vi "Dataset_Reader(Classification).vi"(3 "Train dataset path":path=path "D:/working/Anomaly Detection/Train") -> (0 "error out":errorcluster, 1 "Dataset":T1)   [LabVIEW 2020]
uses:
  <vilib>/Ngene/DeepLTK/Toolkit/NN_Data/API/DataSet_Types/NN_DataSet(In1D_Out1D).ctl
  <vilib>/Ngene/DeepLTK/Toolkit/NN_Data/API/DataRef_Types/NN_Data_ref(2D_SGL).ctl
  <vilib>/Ngene/DeepLTK/Toolkit/NN_Data/API/DataRef_Types/NN_Data_ref(1D_I32).ctl
  8703a7eb-7e7a-4f89-999d-626aab8b5f58.vi
  <vilib>/Utility/file.llb/Read Delimited Spreadsheet (DBL).vi
  <vilib>/Comparison/Less/Less Functor/Less Functor.lvclass
  <vilib>/Ngene/DeepLTK/Toolkit/Deep_Learning_Toolkit_by_Ngene.lvlib
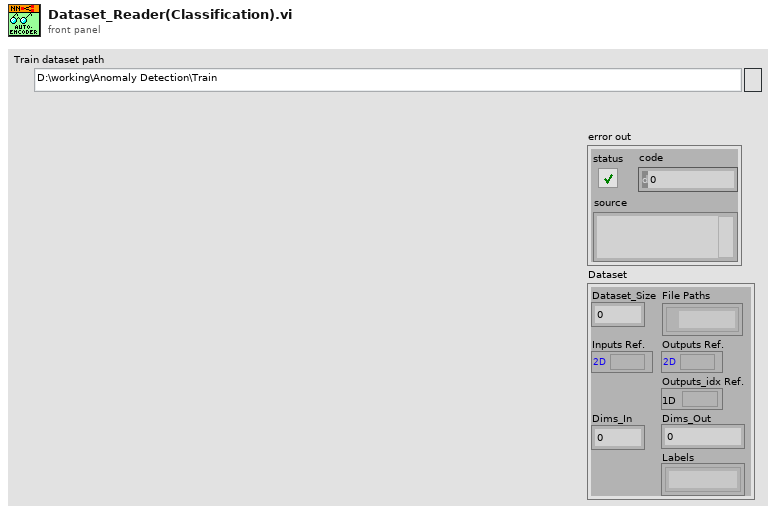
[diagram p1: front panel]
types:
  T1 = typedef "Deep_Learning_Toolkit_by_Ngene.lvlib/NN_DataSet(In1D_Out1D).ctl" = cluster{"Inputs Ref.":T2, "Outputs Ref.":T2, "Dims_In":i32, "Dataset_Size":i32, "Outputs_idx Ref.":T3, "Dims_Out":i32, "Labels":string[], "File Paths":path[]}
  T2 = typedef "Deep_Learning_Toolkit_by_Ngene.lvlib/NN_Data_ref(2D_SGL).ctl" = refnum<data-value>
  T3 = typedef "Deep_Learning_Toolkit_by_Ngene.lvlib/NN_Data_ref(1D_I32).ctl" = refnum<data-value>
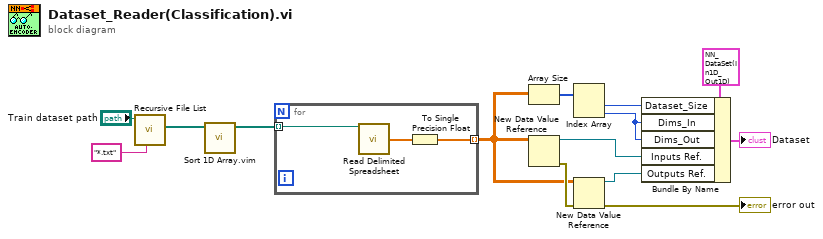
[diagram p0: block diagram]
diagram:
  n1 = call <vilib>:"Recursive File List.vi"("pattern"="*.txt", "Folder Path"="Train dataset path") -> ("All Files in Dir"=w6:path[])  [unwired: 5 in, 4 out]
  n2 = call "Sort 1D Array.vim"("unsorted array"=w6) -> ("sorted array"=w3:path[])  [unwired: 10 in]
  n3 = for {
    tunnel: w3 -> [w17] mode=indexing
    tunnel: [w15] -> w5 mode=indexing
    n4 = call-poly <vilib>:"Read Delimited Spreadsheet.vi"("file path (dialog if empty)"=w17) -> ("first row"=w16:dbl[])  [unwired: 9 in, 5 out]
    n5 = To Single Precision Float(number=w16) -> (single precision float=w15:sgl[])
  }
  n6 = Array Size(array=w5) -> (size(s)=w12:i32[])
  n7 = New Data Value Reference(data value=w5) -> (data value reference=w14:refnum<data-value>, error out=w11:errorcluster)  [unwired: 1 in]
  n8 = Index Array(array=w12) -> (element #1=w10:i32, element #2=w9:i32)  [unwired: 2 in]
  n9 = New Data Value Reference(data value=w5, error in=w11) -> (data value reference=w13:refnum<data-value>, error out=→"error out":errorcluster)
  n10 = Bundle By Name(cluster=T1 {"Inputs Ref."=refnum, "Outputs Ref."=refnum, "Dims_In"=0, "Dataset_Size"=0, "Outputs_idx Ref."=refnum, "Dims_Out"=0, "Labels"=[], "File Paths"=[]} ("Dataset(In1D_Out1D)"), "Dataset_Size"=w10, "Dims_In"=w9, "Dims_Out"=w9, "Inputs Ref."=w14, "Outputs Ref."=w13) -> (→"Dataset":T1)
